vi "Vision Processing.vi"(4 "error in (no error)":errorcluster, 7 "Image Size":T1=enum."320x240") -> ()   [LabVIEW 2016]
doc: "This VI runs in parallel to other tasks. It gets images from the camera, processes them for color or shape and use that information to affect robot behavior."
uses:
  <vilib>/Rock Robotics/WPI/Camera/WPI_CameraImageSize.ctl
  <vilib>/Rock Robotics/WPI/Camera/WPI_CameraWhite Balance Values.ctl
  <vilib>/Rock Robotics/WPI/Camera/WPI_CameraExposure Values.ctl
  <vilib>/Rock Robotics/WPI/Camera/WPI_CameraFrameRate.ctl
  Robot Global Data.vi
  LabVIEW Data/Zeus Dashboard/VisionProcessingBoolean.vi
  <vilib>/Rock Robotics/Network Tables/NT Read Number.vi
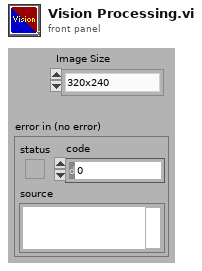
[diagram p1: front panel]
types:
  T1 = typedef "WPI_CameraImageSize.ctl" = enum16{"640x480", "320x240", "160x120", "Custom"}
  T2 = typedef "WPI_CameraFrameRate.ctl" = u32
  T3 = typedef "WPI_CameraExposure Values.ctl" = enum16{"Auto", "Flicker-free 50 Hz", "Flicker-free 60 Hz", "Hold current", "Custom"}
  T4 = typedef "WPI_CameraWhite Balance Values.ctl" = enum16{"Auto", "Fixed indoor", "Fixed outdoor 1", "Fixed outdoor 2", "Fixed fluorescent 1", "Fixed fluorescent 2", "Hold current", "Custom"}
  T5 = typedef "Image Type" = u32
  T6 = typedef "WPI_CameraDevRef.ctl" = cluster{"Camera Address":string, "CameraStatus":errorcluster}
  T7 = typedef "IMAQ Image.ctl" = refnum<image>
  T8 = cluster{"Position":cluster{"x":sgl, "y":sgl}, "Angle":sgl, "Scale":sgl, "Score":sgl, "Bounding Box":cluster{"x":sgl, "y":sgl}[]}[]
  T9 = cluster{"Position":cluster{"x":sgl, "y":sgl}, "Angle":sgl, "Scale":sgl, "Score":sgl, "Bounding Box":cluster{"x":sgl, "y":sgl}[]}
  T10 = typedef "WPI_DigitalOutputDevRef.ctl" = cluster{"DIO Channel":T11, "DevStatus":errorcluster}
  T11 = typedef "FPGA_DIOChannel.ctl" = enum8{"DIO 0", "DIO 1", "DIO 2", "DIO 3", "DIO 4", "DIO 5", "DIO 6", "DIO 7", "DIO 8", "DIO 9", "DIO MXP 0", "DIO MXP 1", "DIO MXP 2", "DIO MXP 3", "DIO MXP 4", "DIO MXP 5", "DIO MXP 6", "DIO MXP 7", "DIO MXP 8", "DIO MXP 9", "DIO MXP 10", "DIO MXP 11", "DIO MXP 12", "DIO MXP 13", "DIO MXP 14", "DIO MXP 15", "SPI Port CS1", "SPI Port CS2", "SPI Port CS3", "SPI Port MISO", "SPI Port MOSI", "Invalid"}
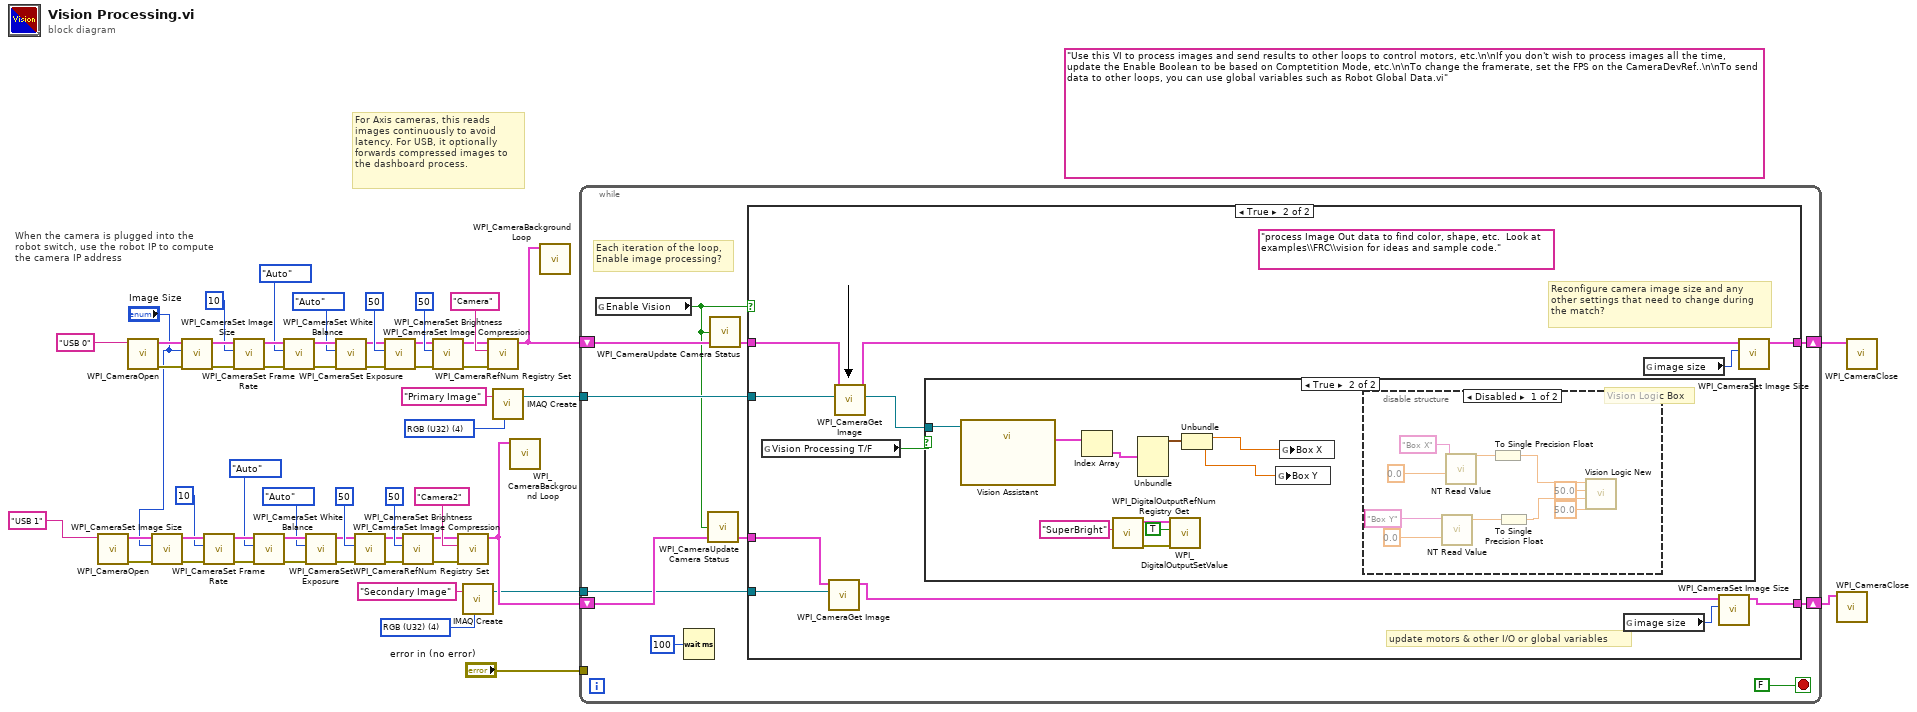
[diagram p0: block diagram]
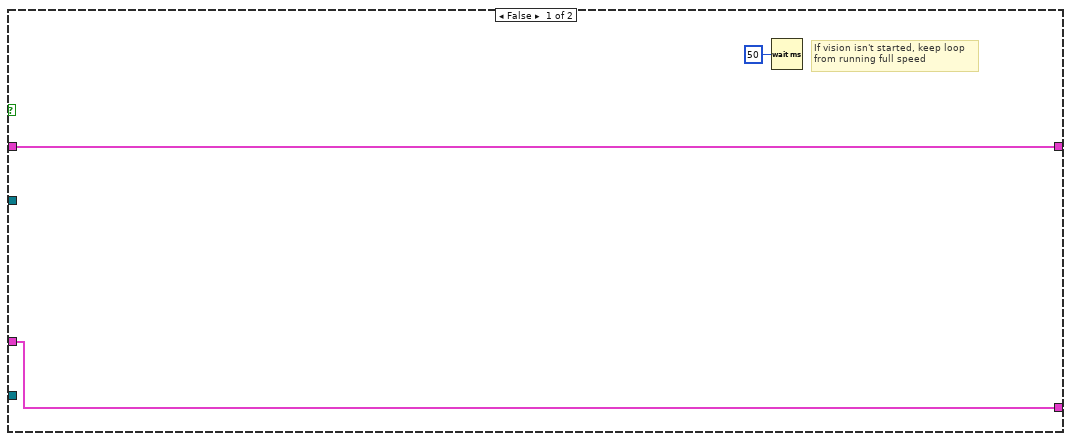
[diagram p2: hidden frame]
diagram:
  w28 = T5 4 items=["Grayscale (U8)", "Grayscale (I16)", "Grayscale (SGL)", "Complex (CSG)", "RGB (U32)", "HSL (U32)", "RGB (U64)"] ("Image Type")
  (unwired) "Use this VI to process images and send results to other loops to control motors, etc.\n\nIf you don't wish to process images all the time, update the Enable Boolean to be based on Comptetition Mode, etc.\n\nTo change the framerate, set the FPS on the CameraDevRef..\n\nTo send data to other loops, you can use global variables such as Robot Global Data.vi"
  w54 = T5 4 items=["Grayscale (U8)", "Grayscale (I16)", "Grayscale (SGL)", "Complex (CSG)", "RGB (U32)", "HSL (U32)", "RGB (U64)"] ("Image Type")
  # "When the camera is plugged into the\nrobot switch, use the robot IP to compute\nthe camera IP address"
  # "For Axis cameras, this reads\nimages continuously to avoid\nlatency. For USB, it optionally\nforwards compressed images to\nthe dashboard process."
  n1 = call <vilib>:"WPI_CameraOpen.vi"("Camera Address"="USB 1" ("format string")) -> ("error out"=w17:errorcluster, "CameraDevRef"=w18:T6)  [unwired: 1 in, 8 out]
  n2 = call <vilib>:"WPI_CameraOpen.vi"("Camera Address"="USB 0" ("format string")) -> ("error out"=w42:errorcluster, "CameraDevRef"=w43:T6)  [unwired: 1 in, 8 out]
  n3 = call <vilib>:"WPI_CameraSet Image Size.vi"("error in (no error)"=w17, "Image Size"="Image Size", "CameraDevRef"=w18) -> ("error out"=w16:errorcluster, "CameraDevRef Out"=w19:T6)  [unwired: 1 in, 6 out]
  n4 = call <vilib>:"WPI_CameraSet Image Size.vi"("error in (no error)"=w42, "Image Size"="Image Size", "CameraDevRef"=w43) -> ("error out"=w41:errorcluster, "CameraDevRef Out"=w44:T6)  [unwired: 1 in, 6 out]
  n5 = call <vilib>:"WPI_CameraSet Frame Rate.vi"("error in (no error)"=w16, "Frame Rate (fps)"=T2 10, "CameraDevRef"=w19) -> ("error out"=w15:errorcluster, "CameraDevRef Out"=w21:T6)  [unwired: 7 out]
  n6 = call <vilib>:"WPI_CameraSet Frame Rate.vi"("error in (no error)"=w41, "Frame Rate (fps)"=T2 10, "CameraDevRef"=w44) -> ("error out"=w40:errorcluster, "CameraDevRef Out"=w46:T6)  [unwired: 7 out]
  n7 = call <vilib>:"WPI_CameraSet White Balance.vi"("error in (no error)"=w15, "White Balance"=WPI_CameraWhite_Balance_Values."Auto", "CameraDevRef"=w21) -> ("error out"=w14:errorcluster, "CameraDevRef Out"=w20:T6)  [unwired: 1 in, 6 out]
  n8 = call <vilib>:"WPI_CameraSet White Balance.vi"("error in (no error)"=w40, "White Balance"=WPI_CameraWhite_Balance_Values."Auto", "CameraDevRef"=w46) -> ("error out"=w39:errorcluster, "CameraDevRef Out"=w45:T6)  [unwired: 1 in, 6 out]
  n9 = call <vilib>:"WPI_CameraSet Exposure.vi"("error in (no error)"=w14, "Exposure"=WPI_CameraExposure_Values."Auto", "CameraDevRef"=w20) -> ("error out"=w13:errorcluster, "CameraDevRef Out"=w23:T6)  [unwired: 1 in, 6 out]
  n10 = call <vilib>:"WPI_CameraSet Exposure.vi"("error in (no error)"=w39, "Exposure"=WPI_CameraExposure_Values."Auto", "CameraDevRef"=w45) -> ("error out"=w38:errorcluster, "CameraDevRef Out"=w48:T6)  [unwired: 1 in, 6 out]
  n11 = call <vilib>:"WPI_CameraSet Image Compression.vi"("error in (no error)"=w13, "Compression"=50, "CameraDevRef"=w23) -> ("error out"=w12:errorcluster, "CameraDevRef Out"=w22:T6)  [unwired: 7 out]
  n12 = call <vilib>:"WPI_CameraSet Image Compression.vi"("error in (no error)"=w38, "Compression"=50, "CameraDevRef"=w48) -> ("error out"=w37:errorcluster, "CameraDevRef Out"=w47:T6)  [unwired: 7 out]
  n13 = call <vilib>:"WPI_CameraSet Brightness.vi"("error in (no error)"=w12, "Brightness"=50, "CameraDevRef"=w22) -> ("error out"=w10:errorcluster, "CameraDevRef Out"=w11:T6)  [unwired: 7 out]
  n14 = call <vilib>:"WPI_CameraSet Brightness.vi"("error in (no error)"=w37, "Brightness"=50, "CameraDevRef"=w47) -> ("error out"=w35:errorcluster, "CameraDevRef Out"=w36:T6)  [unwired: 7 out]
  n15 = call <vilib>:"WPI_CameraRefNum Registry Set.vi"("error in (no error)"=w10, "refnum name"="Camera2", "CameraDevRef"=w11) -> ("CameraDevRef"=w6:T6)  [unwired: 1 in, 7 out]
  n16 = call "IMAQ Create"("Image Name"="Secondary Image", "Image Type"=w28) -> ("New Image"=w5:T7)  [unwired: 2 in, 2 out]
  n17 = call <vilib>:"WPI_CameraRefNum Registry Set.vi"("error in (no error)"=w35, "refnum name"="Camera", "CameraDevRef"=w36) -> ("CameraDevRef"=w31:T6)  [unwired: 1 in, 7 out]
  n18 = call "IMAQ Create"("Image Name"="Primary Image", "Image Type"=w54) -> ("New Image"=w52:T7)  [unwired: 2 in, 2 out]
  n19 = call <vilib>:"WPI_CameraBackground Loop.vi"("CameraDevRef"=w6) -> ()  [unwired: 11 in]
  n20 = call <vilib>:"WPI_CameraBackground Loop.vi"("CameraDevRef"=w31) -> ()  [unwired: 11 in]
  n21 = while {
    shift-right: [w64] -> w30
    shift-left: w31 -> [w62]
    tunnel: w52 -> [w63]
    tunnel: "error in (no error)" -> [_]
    tunnel: w5 -> [w56]
    shift-right: [w55] -> w4
    shift-left: w6 -> [w59]
    stop <- FALSE stop-if-true
    # "Each iteration of the loop,\nEnable image processing?"
    n22 = global read "Robot Global Data.vi" "Enable Vision"() -> (w58:bool)
    n23 = Wait (ms)(milliseconds to wait=u32 100) -> ()  [unwired: 1 out]
    n24 = call <vilib>:"WPI_CameraUpdate Camera Status.vi"("CameraDevRef In"=w59, "Enable Vision"=w58) -> ("CameraDevRef Out"=w57:T6)  [unwired: 3 in]
    n25 = call <vilib>:"WPI_CameraUpdate Camera Status.vi"("CameraDevRef In"=w62, "Enable Vision"=w58) -> ("CameraDevRef Out"=w61:T6)  [unwired: 3 in]
    n26 = case shown="True" w58 {
      tunnel: w63 -> [_ w79]
      tunnel: [w68 w80] -> w64
      tunnel: w61 -> [w68 w77]
      tunnel: w57 -> [w66 w73]
      tunnel: w56 -> [_ w72]
      tunnel: [w66 w69] -> w55
      frame False {
        # "If vision isn't started, keep loop\nfrom running full speed"
        n27 = Wait (ms)(milliseconds to wait=u32 50) -> ()  [unwired: 1 out]
      }
      frame True {
        (unwired) "process Image Out data to find color, shape, etc.  Look at examples\\FRC\\vision for ideas and sample code."
        # "update motors & other I/O or global variables"
        # "Reconfigure camera image size and any\nother settings that need to change during\nthe match?"
        n28 = global read "VisionProcessingBoolean.vi" "Vision Processing T/F"() -> (w75:bool)
        n29 = call <vilib>:"WPI_CameraGet Image.vi"("Image"=w72, "CameraDevRef"=w73) -> ("CameraDevRef Out"=w70:T6)  [unwired: 1 in, 8 out]
        n30 = call <vilib>:"WPI_CameraGet Image.vi"("Image"=w79, "CameraDevRef"=w77) -> ("Image Out"=w74:T7, "CameraDevRef Out"=w76:T6)  [unwired: 1 in, 7 out]
        n31 = case shown="True" w75 {
          tunnel: w74 -> [_ w82]
          frame False {
          }
          frame True {
            # "Vision Logic Box"
            n32 = call "Vision Assistant"("Image In"=w82) -> ("Calibrated Matches (Pattern Matching 1)"=w81:T8)  [unwired: 24 in, 2 out]
            n33 = Index Array(array=w81) -> (element=w90:T9)  [unwired: 1 in]
            n34 = call <vilib>:"WPI_DigitalOutputRefNum Registry Get.vi"("refnum name"="SuperBright") -> ("error out"=w87:errorcluster, "DigitalOutputDevRef"=w86:T10)  [unwired: 9 in]
            n35 = Unbundle(w90) -> ("Position"=w89:cluster{"x":sgl, "y":sgl})  [unwired: 4 out]
            n36 = call <vilib>:"WPI_DigitalOutputSetValue.vi"("error in (no error)"=w87, "Value"=TRUE, "DigitalOutputDevRef"=w86) -> ()  [unwired: 7 in, 2 out]
            n37 = Unbundle(w89) -> ("x"=w84:sgl, "y"=w83:sgl)
            n38 = global write "VisionProcessingBoolean.vi" "Box Y"(w83) -> ()
            n39 = global write "VisionProcessingBoolean.vi" "Box X"(w84) -> ()
            n40 = disable-structure shown="Disabled" {
              frame Disabled {
                n41 = call-poly <vilib>:"NT Read Value.vi"("Default Value"=0.0, "Name"="Box Y") -> ("Numeric"=w93:dbl)  [unwired: 8 in, 1 out]
                n42 = call-poly <vilib>:"NT Read Value.vi"("Default Value"=0.0, "Name"="Box X") -> ("Numeric"=w91:dbl)  [unwired: 8 in, 1 out]
                n43 = To Single Precision Float(number=w91) -> (single precision float=w92:sgl)
                n44 = To Single Precision Float(number=w93) -> (single precision float=w94:sgl)
                n45 = call "Vision Logic New.vi"("Y Default/Base Value"=sgl 50.0, "Y Coordinate of the Box"=w94, "X Default/Base Value"=sgl 50.0, "X Coordinate of the Box"=w92) -> ()  [unwired: 8 in]
              }
              frame Enabled {
              }
            }
          }
        }
        n46 = global read "Robot Global Data.vi" "image size"() -> (w71:T1)
        n47 = global read "Robot Global Data.vi" "image size"() -> (w78:T1)
        n48 = call <vilib>:"WPI_CameraSet Image Size.vi"("Image Size"=w71, "CameraDevRef"=w70) -> ("CameraDevRef Out"=w69:T6)  [unwired: 2 in, 7 out]
        n49 = call <vilib>:"WPI_CameraSet Image Size.vi"("Image Size"=w78, "CameraDevRef"=w76) -> ("CameraDevRef Out"=w80:T6)  [unwired: 2 in, 7 out]
      }
    }
  }
  n50 = call <vilib>:"WPI_CameraClose.vi"("CameraDevRef"=w4) -> ()  [unwired: 1 in, 10 out]
  n51 = call <vilib>:"WPI_CameraClose.vi"("CameraDevRef"=w30) -> ()  [unwired: 1 in, 10 out]
